vi "GeraSinalAM.vi"(0 "params":variant, 2 "Tx Aquisicao":dbl, 5 "estadoIn":variant) -> (15 "sinal":waveform(dbl), 19 "estadoOut":variant)   [LabVIEW 2017]
uses:
  Typedefs/Tipo_ParamsAMgen.ctl
  Typedefs/Tipo_ComponenteSinalRuidoComposto.ctl
  Typedefs/Tipo_TipoSinalCarrier.ctl
  <vilib>/Analysis/NI_AALBase.lvlib
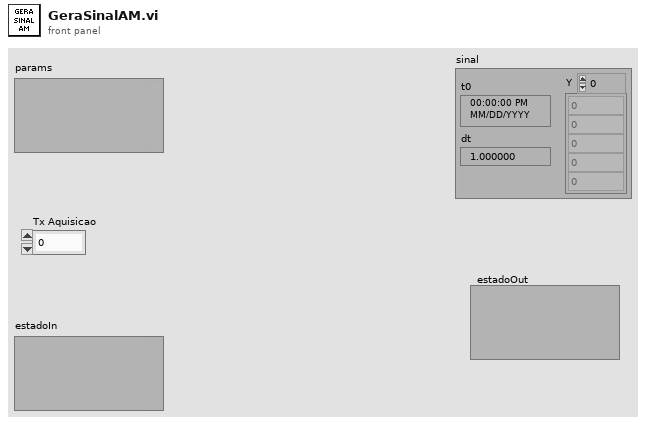
[diagram p1: front panel]
types:
  T1 = typedef "Tipo_ParamsAMgen.ctl" = cluster{"Componentes":T2[], "Carrier Frequency":dbl, "Modulation":dbl, "Ruído Total":dbl, "Tipo":T3}
  T2 = typedef "Tipo_ComponenteSinalRuidoComposto.ctl" = cluster{"Amplit.: ":dbl, "Freq. (Hz): ":dbl, "Fase (º):":dbl, "Ruido":dbl}
  T3 = typedef "Tipo_TipoSinalCarrier.ctl" = enum16{"Ruído", "Senóide"}
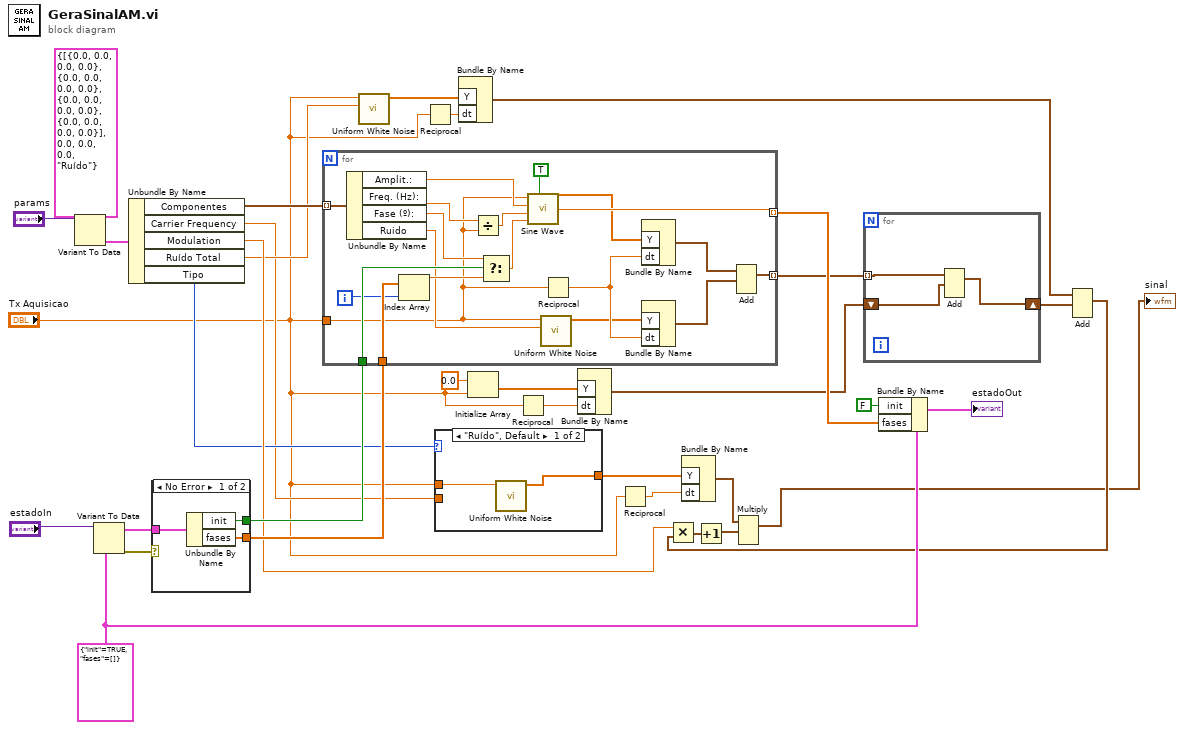
[diagram p0: block diagram]
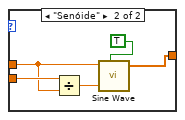
[diagram p2: hidden frame]
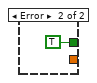
[diagram p3: hidden frame]
diagram:
  w25 = cluster{"init":bool, "fases":dbl[]} {"init"=TRUE, "fases"=[]}
  n1 = Variant To Data(type=T1 {"Componentes"=[{"Amplit.: "=0.0, "Freq. (Hz): "=0.0, "Fase (º):"=0.0, "Ruido"=0.0}, {"Amplit.: "=0.0, "Freq. (Hz): "=0.0, "Fase (º):"=0.0, "Ruido"=0.0}, {"Amplit.: "=0.0, "Freq. (Hz): "=0.0, "Fase (º):"=0.0, "Ruido"=0.0}, {"Amplit.: "=0.0, "Freq. (Hz): "=0.0, "Fase (º):"=0.0, "Ruido"=0.0}], "Carrier Frequency"=0.0, "Modulation"=0.0, "Ruído Total"=0.0, "Tipo"=enum."Ruído"} ("Cluster"), Variant="params") -> (data=w32:T1)  [unwired: 1 in, 1 out]
  n2 = Variant To Data(type=w25, Variant="estadoIn") -> (data=w29:cluster{"init":bool, "fases":dbl[]}, error out=w26:errorcluster)  [unwired: 1 in]
  n3 = Unbundle By Name(w32) -> ("Componentes"=w31:T2[], "Carrier Frequency"=w4:dbl, "Modulation"=w9:dbl, "Ruído Total"=w8:dbl, "Tipo"=w5:T3)
  n4 = case shown="No Error" w26 {
    tunnel: w29 -> [w37 _]
    tunnel: [w36 TRUE ("init")] -> w28
    tunnel: [w35 _] -> w27
    frame No Error {
      n5 = Unbundle By Name(w37) -> ("init"=w36:bool, "fases"=w35:dbl[])
    }
    frame Error {
    }
  }
  n6 = for {
    tunnel: w31 -> [w52] mode=indexing
    tunnel: w28 -> [w57]
    tunnel: w27 -> [w54]
    tunnel: [w53] -> w22 mode=indexing
    tunnel: "Tx Aquisicao" -> [w44]
    tunnel: [w39] -> w21 mode=indexing
    i -> [w47]
    n7 = Unbundle By Name(w52) -> ("Amplit.:"=w51:dbl, "Freq. (Hz):"=w50:dbl, "Fase (º):"=w49:dbl, "Ruido"=w45:dbl)
    n8 = Index Array(array=w54, index=w47) -> (element=w48:dbl)
    n9 = Divide(x=w50, y=w44) -> (x/y=w58:dbl)
    n10 = Select(t=w49, s=w57, f=w48) -> (s? t:f=w56:dbl)
    n11 = call <vilib>:"Sine Wave.vi"("samples"=w44, "amplitude"=w51, "frequency"=w58, "phase in"=w56, "reset phase"=TRUE) -> ("sine wave"=w46:dbl[], "phase out"=w53:dbl)  [unwired: 1 out]
    n12 = call <vilib>:"Uniform White Noise.vi"("amplitude"=w45, "samples"=w44) -> ("uniform white noise"=w42:dbl[])  [unwired: 8 in, 1 out]
    n13 = Reciprocal(x=w44) -> (1/x=w43:dbl)
    n14 = Bundle By Name("Y"=w46, "dt"=w43) -> (w40:waveform(dbl))  [unwired: 1 in]
    n15 = Bundle By Name("Y"=w42, "dt"=w43) -> (w41:waveform(dbl))  [unwired: 1 in]
    n16 = Add(1:w41, 2:w40) -> (0:w39:waveform(dbl))  [unwired: 1 in, 1 out]
  }
  n17 = call <vilib>:"Uniform White Noise.vi"("amplitude"=w8, "samples"="Tx Aquisicao") -> ("uniform white noise"=w19:dbl[])  [unwired: 8 in, 1 out]
  n18 = Reciprocal(x="Tx Aquisicao") -> (1/x=w18:dbl)
  n19 = case shown="\"Ruído\", Default" w5 {
    tunnel: "Tx Aquisicao" -> [w60 w62]
    tunnel: w4 -> [_ w64]
    tunnel: [w59 w61] -> w1
    frame "Ruído", Default {
      n20 = call <vilib>:"Uniform White Noise.vi"("samples"=w60) -> ("uniform white noise"=w59:dbl[])  [unwired: 9 in, 1 out]
    }
    frame "Senóide" {
      n21 = Divide(x=w64, y=w62) -> (x/y=w65:dbl)
      n22 = call <vilib>:"Sine Wave.vi"("samples"=w62, "frequency"=w65, "reset phase"=TRUE) -> ("sine wave"=w61:dbl[])  [unwired: 2 in, 2 out]
    }
  }
  n23 = Bundle By Name("Y"=w19, "dt"=w18) -> (w17:waveform(dbl))  [unwired: 1 in]
  n24 = Initialize Array(0.0 ("element"), "Tx Aquisicao") -> (w15:dbl[])
  n25 = Reciprocal(x="Tx Aquisicao") -> (1/x=w14:dbl)
  n26 = Bundle By Name("Y"=w15, "dt"=w14) -> (w13:waveform(dbl))  [unwired: 1 in]
  n27 = Reciprocal(x="Tx Aquisicao") -> (1/x=w2:dbl)
  n28 = Bundle By Name("Y"=w1, "dt"=w2) -> (w7:waveform(dbl))  [unwired: 1 in]
  n29 = for {
    tunnel: w21 -> [w68] mode=indexing
    shift-right: [w66] -> w20
    shift-left: w13 -> [w67]
    n30 = Add(1:w67, 2:w68) -> (0:w66:waveform(dbl))  [unwired: 1 in, 1 out]
  }
  n31 = Bundle By Name(cluster=w25, "init"=FALSE, "fases"=w22) -> (→"estadoOut":cluster{"init":bool, "fases":dbl[]})
  n32 = Add(1:w20, 2:w17) -> (0:w10:waveform(dbl))  [unwired: 1 in, 1 out]
  n33 = Multiply(x=w9, y=w10) -> (x*y=w12:waveform(dbl))
  n34 = Increment(x=w12) -> (x+1=w11:waveform(dbl))
  n35 = Multiply(1:w11, 2:w7) -> (0:→"sinal":waveform(dbl))  [unwired: 1 in, 1 out]
